vi "Main-PSD+EQP_YCC.vi"() -> ()   [LabVIEW 2014]
uses:
  Main-Stage-Based/(Global) Current handle and LaserPower_YCC.vi
  <vilib>/DAQmx/create/channels.llb/DAQmx Create Channel (AI-Voltage-Basic).vi
  <vilib>/DAQmx/configure/timing.llb/DAQmx Timing (Sample Clock).vi
  <vilib>/DAQmx/read.llb/DAQmx Read (Analog 2D DBL NChan NSamp).vi
panel:
  out "QPD raw(V) xyz":dbl[][](array[numeric])
  out "kx (pN/nm)":dbl
  in  "Who's Data":enum16{"YCC", "PYW", "LCH", "YYH"}(ring)
  in  "Save?":bool
  out "Frequency (Hz)\n0,df, 2df,...(n/2-1)Fs":dbl[](array[numeric])
  in  "Temperature (C)":dbl=22.0
  out "df (freq. resolution) Hz":dbl
  in  "record time per cycle (s)":dbl=0.125
  in  "EQP on?":bool
  out "Beta (V/um)":dbl[](array[numeric])
  out "Varicance (V^2)":dbl[](array[numeric])
  out "y-variance (V)":dbl format="%0.2f"
  out "x-variance (V)":dbl format="%0.2f"
  out "Y-conversion factor (V/um)":dbl
  out "X-conversion factor (V/um)":dbl
  out "EQP-Trap Stiffness (pN/nm)":dbl[](array[numeric])
  out "best fit parameters-y":dbl[](array[numeric])
  out "best fit parameters-z":dbl[](array[numeric])
  out "best fit parameters-x":dbl[](array[numeric])
  in  "Fit z?":bool
  in  "Fit y?":bool
  out "best nonlinear fit PSDz":dbl[](array[numeric])
  out "best nonlinear fit PSDy":dbl[](array[numeric])
  out "best nonlinear fit PSDx":dbl[](array[numeric])
  in  "Custum Fs (Hz)":i32
  in  "Focal shift factor":dbl=1.22
  out "best fit parameters":dbl[][](array[numeric])
  out "kx/kz":dbl
  in  "Freq End Cut":dbl=60000.0
  in  "Freq Strat Cut":dbl=10.0
  out "Trap Stiffness (pN/nm)":dbl[](array[numeric])
  in  "bead height (um)":dbl=2.0
  in  "bead radius (um)":dbl=0.515
  out "PSDz":dbl[](array[numeric])
  out "PSDy":dbl[](array[numeric])
  out "PSDx":dbl[](array[numeric])
  out "Frequency (Hz)\n0,df, 2df,...1/2Fs":dbl[](array[numeric])
  in  "Tab Control":enum32{"PSD x & y", "PSD x & z"}(tab)
  out "PSD x & y":T1(graph)
  out "PSD x & z":T2(graph)
  out "Corner Frequency (Hz)\n(fx,fy,fz)":dbl[](array[numeric])
  in  "Fit Lorentz PSD?":bool=TRUE
  out "Avg. PSD":dbl[][](array[numeric])
  out "# of PSD sum":i32
  in  "# of PSD Avg.":dbl=50.0
  in  "stop to fit":bool
  in  "T=NI made PSD\nF=YCC made PSD":bool
  out "Sampling rate (Hz)":i32
  in  "physical channels":tag="Dev2/ai2, Dev2/ai0, Dev2/ai16"
  in  "Sampling Rate (Hz)":T3(ring)=enum."131072"
  # "Fc=80k for fs=131072Hz"
  # "x"
  # "y"
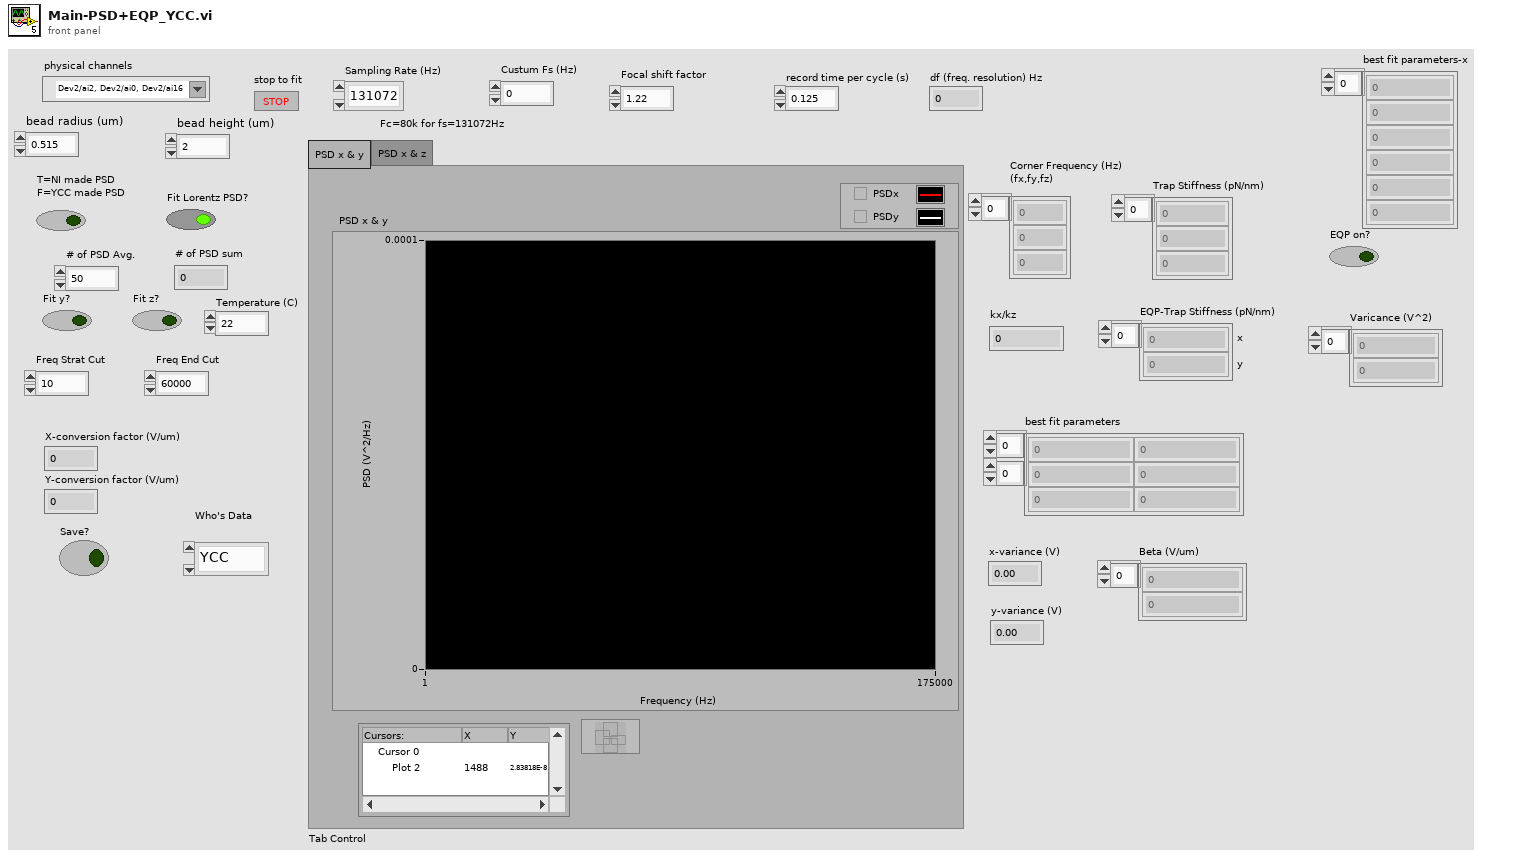
[diagram p1: front panel]
types:
  T1 = cluster{"Frequency (Hz)\ndf, 2df,...1/2Fs":dbl[], "PSDy":dbl[]}[]
  T2 = cluster{"Frequency (Hz)\ndf, 2df,...1/2Fs":dbl[], "PSDz":dbl[]}[]
  T3 = enum16{"custum", "16384", "32768", "65536", "131072", "262144"}
  T4 = cluster{"Frequency (Hz)\n0,df, 2df,...1/2Fs":dbl[], "PSDx":dbl[]}
  T5 = cluster{"Frequency (Hz)\n0,df, 2df,...1/2Fs":dbl[], "PSDz":dbl[]}
  T6 = cluster{"Frequency (Hz)\n0,df, 2df,...1/2Fs":dbl[], "PSDy":dbl[]}
  T7 = cluster{"Frequency (Hz)\n0,df, 2df,...1/2Fs":dbl[], "PSDz":dbl[]}[]
  T8 = cluster{"Frequency (Hz)\n0,df, 2df,...1/2Fs":dbl[], "PSDy":dbl[]}[]
  T9 = cluster{"Frequency (Hz)\n0,df, 2df,...1/2Fs":dbl[], "best nonlinear fit PSDz":dbl[]}
  T10 = cluster{"Frequency (Hz)\n0,df, 2df,...1/2Fs":dbl[], "best nonlinear fit PSDx":dbl[]}
  T11 = cluster{"Frequency (Hz)\n0,df, 2df,...1/2Fs":dbl[], "best nonlinear fit PSDy":dbl[]}
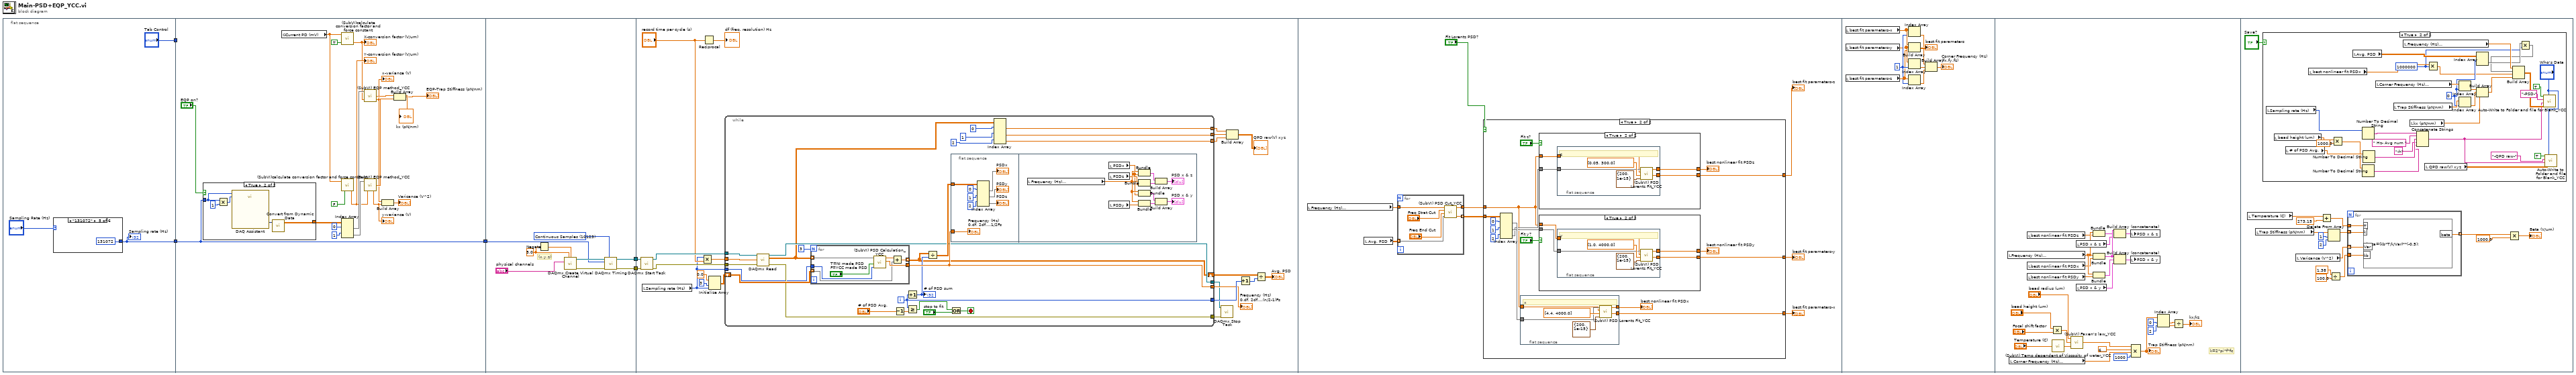
[diagram p0: block diagram]
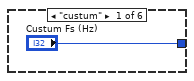
[diagram p2: hidden frame]
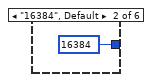
[diagram p3: hidden frame]
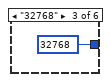
[diagram p4: hidden frame]
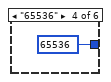
[diagram p5: hidden frame]
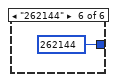
[diagram p6: hidden frame]
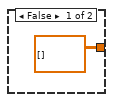
[diagram p7: hidden frame]
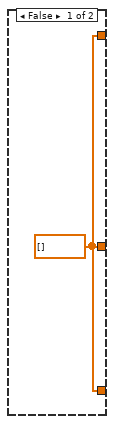
[diagram p8: hidden frame]
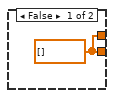
[diagram p9: hidden frame]
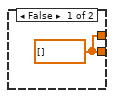
[diagram p10: hidden frame]
diagram:
  n1 = flat-sequence {
    tunnel: [w7] -> w3
    tunnel: ["Tab Control"] -> w1
    tunnel: w3 -> [w32]
    tunnel: [w32] -> w2
    tunnel: w1 -> [_]
    tunnel: w2 -> [w45]
    tunnel: [w42] -> w5
    tunnel: [w41] -> w4
    tunnel: w5 -> [w69]
    tunnel: w4 -> [w68]
    frame #0 {
      n2 = case shown="\"131072\"" "Sampling Rate (Hz)" {
        tunnel: ["Custum Fs (Hz)" 16384 32768 65536 131072 262144] -> w7
        frame "custum" {
        }
        frame "16384", Default {
        }
        frame "32768" {
        }
        frame "65536" {
        }
        frame "131072" {
        }
        frame "262144" {
        }
      }
      "Sampling rate (Hz)" <- w7
    }
    frame #1 {
      n3 = case shown="True" "EQP on?" {
        tunnel: w32 -> [_ w38]
        tunnel: [dbl[][] [] ("Array") w34] -> w21
        frame False {
        }
        frame True {
          n4 = Multiply(x=w38, y=1) -> (x*y=w36:i32)
          n5 = call "DAQ Assistant"("rate"=w38, "number of samples"=w36) -> ("data"=w35:dynamicdata)  [unwired: 15 in, 2 out]
          n6 = call "Convert from Dynamic Data"("Dynamic Data Type"=w35) -> ("Array"=w34:dbl[][])  [unwired: 3 in]
        }
      }
      n7 = global read "(Global) Current handle and LaserPower_YCC.vi" "Current PD (mV)"() -> (w18:dbl)
      n8 = Index Array(array=w21, index (row) #1=0 ("index (row)"), index (row) #2=1 ("index (row)")) -> (element #1=w29:dbl[], element #2=w28:dbl[])  [unwired: 2 in]
      n9 = call "(SubVI)calculate conversion factor and force constant.vi"("X=T\nY=F"=TRUE ("X=T\nY=F"), "laser power (mW)"=w18) -> ("conversion factor (V/um)"=w17:dbl)  [unwired: 2 in, 1 out]
      "X-conversion factor (V/um)" <- w17
      n10 = call "(SubVI)calculate conversion factor and force constant.vi"("X=T\nY=F"=FALSE ("X=T\nY=F"), "laser power (mW)"=w18) -> ("conversion factor (V/um)"=w19:dbl)  [unwired: 2 in, 1 out]
      "Y-conversion factor (V/um)" <- w19
      n11 = call "(SubVI) EQP method_YCC.vi"("Sensitivity (V/um)"=w17, "position (V)"=w29) -> ("variance (V)"=w24:dbl, "k (pN/nm)"=w27:dbl)  [unwired: 2 in]
      "x-variance (V)" <- w24
      "kx (pN/nm)" <- w27
      n12 = call "(SubVI) EQP method_YCC.vi"("Sensitivity (V/um)"=w19, "position (V)"=w28) -> ("variance (V)"=w23:dbl, "k (pN/nm)"=w26:dbl)  [unwired: 2 in]
      "y-variance (V)" <- w23
      n13 = Build Array(w24, w23) -> (→"Varicance (V^2)":dbl[])
      n14 = Build Array(w27, w26) -> (→"EQP-Trap Stiffness (pN/nm)":dbl[])
    }
    frame #2 {
      w40 = 5.0 ("maximum value")
      w43 = 10123 items=["Finite Samples"=10178, "Continuous Samples"=10123, "Hardware Timed Single Point"=12522] ("sample mode")
      # "(x,y,z)"
      n15 = Negate(x=w40) -> (-x=w39:dbl)
      n16 = call-poly <vilib>:"DAQmx Create Virtual Channel.vi"("maximum value"=w40, "minimum value"=w39, "physical channels"="physical channels") -> ("task out"=w46:refnum<k21>, "error out"=w44:errorcluster)  [unwired: 11 in]
      n17 = call-poly <vilib>:"DAQmx Timing.vi"("task/channels in"=w46, "sample mode"=w43, "rate"=w45, "error in"=w44) -> ("task out"=w42:refnum<k21>, "error out"=w41:errorcluster)  [unwired: 10 in]
    }
    frame #3 {
      n18 = call <vilib>:"DAQmx Start Task.vi"("task/channels in"=w69, "error in"=w68) -> ("task out"=w67:refnum<k21>, "error out"=w66:errorcluster)  [unwired: 12 in]
      n19 = local read "Sampling rate (Hz)"() -> (w52:i32)
      n20 = Multiply(x=w52, y="record time per cycle (s)") -> (x*y=w55:dbl)
      n21 = Reciprocal(x="record time per cycle (s)") -> (1/x=→"df (freq. resolution) Hz":dbl)
      n22 = Initialize Array(0.0 ("element"), 3 ("dimension size"), w52) -> (w63:dbl[][])
      n23 = while {
        tunnel: w67 -> [w94]
        tunnel: w66 -> [w93]
        shift-right: [w79] -> w56
        shift-left: w63 -> [w92]
        tunnel: [w83] -> w59
        tunnel: w55 -> [w78]
        tunnel: [w84] -> w62
        tunnel: [w82] -> w58
        tunnel: [w81] -> w57
        tunnel: w52 -> [w77]
        tunnel: [w72] -> w51 mode=concatenating
        tunnel: [w71] -> w50 mode=concatenating
        tunnel: [w70] -> w49 mode=concatenating
        i -> [w84]
        stop <- w87 stop-if-true
        n24 = call-poly <vilib>:"DAQmx Read.vi"("task/channels in"=w94, "number of samples per channel"=w78, "error in"=w93) -> ("task out"=w82:refnum<k21>, "data"=w76:dbl[][], "error out"=w81:errorcluster)  [unwired: 10 in]
        n25 = for {
          N: 3 -> [_]
          tunnel: w76 -> [w119] mode=indexing
          tunnel: w77 -> [w113]
          tunnel: [w116] -> w83
          tunnel: [w115] -> w79 mode=indexing
          tunnel: w92 -> [w114] mode=indexing
          n26 = call "(SubVI) PSD Calculation_YCC.vi"("sampling frequency (Hz)"=w113, "T=NI made PSD\nF=YCC made PSD"="T=NI made PSD\nF=YCC made PSD", "QPD data"=w119) -> ("Frequency (Hz)\n0,df, 2df,...(n/2-1)Fs"=w116:dbl[], "Power Spectrum (V^2 rms) (V^2/Hz)"=w117:dbl[])  [unwired: 3 in]
          n27 = Add(x=w117, y=w114) -> (x+y=w115:dbl[])
        }
        n28 = Decrement(x="# of PSD Avg.") -> (x-1=w89:dbl)
        n29 = Increment(x=w84) -> (x+1=w80:i32)
        "# of PSD sum" <- w80
        n30 = Greater Or Equal?(x=w84, y=w89) -> (x >= y?=w88:bool)
        n31 = Divide(x=w79, y=w80) -> (x/y=w85:dbl[][])
        n32 = Or(x=w88, y="stop to fit") -> (x .or. y?=w87:bool)
        n33 = flat-sequence {
          tunnel: w85 -> [w99]
          tunnel: w83 -> [w96]
          frame #0 {
            n34 = Index Array(array=w99, index (row) #1=0 ("index (row)"), index (row) #2=1 ("index (row)"), index (row) #3=2 ("index (row)")) -> (element #1=→"PSDx":dbl[], element #2=→"PSDy":dbl[], element #3=→"PSDz":dbl[])  [unwired: 3 in]
            "Frequency (Hz)\n0,df, 2df,...1/2Fs" <- w96
          }
          frame #1 {
            n35 = local read "Frequency (Hz)\n0,df, 2df,...1/2Fs"() -> (w108:dbl[])
            n36 = local read "PSDx"() -> (w103:dbl[])
            n37 = local read "PSDz"() -> (w104:dbl[])
            n38 = local read "PSDy"() -> (w109:dbl[])
            n39 = Bundle("Frequency (Hz)\n0,df, 2df,...1/2Fs"=w108, "PSDx"=w103) -> (w106:T4)  [unwired: 1 in]
            n40 = Bundle("Frequency (Hz)\n0,df, 2df,...1/2Fs"=w108, "PSDz"=w104) -> (w105:T5)  [unwired: 1 in]
            n41 = Bundle("Frequency (Hz)\n0,df, 2df,...1/2Fs"=w108, "PSDx"=w103) -> (w110:T4)  [unwired: 1 in]
            n42 = Bundle("Frequency (Hz)\n0,df, 2df,...1/2Fs"=w108, "PSDy"=w109) -> (w111:T6)  [unwired: 1 in]
            n43 = Build Array(w106, w105) -> (→"PSD x & z":T7)
            n44 = Build Array(w110, w111) -> (→"PSD x & y":T8)
          }
        }
        n45 = Index Array(array=w76, index (row) #1=0 ("index (row)"), index (row) #2=1 ("index (row)"), index (row) #3=2 ("index (row)")) -> (element #1=w72:dbl[], element #2=w71:dbl[], element #3=w70:dbl[])  [unwired: 3 in]
      }
      "Frequency (Hz)\n0,df, 2df,...(n/2-1)Fs" <- w59
      n46 = call <vilib>:"DAQmx Stop Task.vi"("task/channels in"=w58, "error in"=w57) -> ()  [unwired: 12 in, 2 out]
      n47 = Build Array(w51, w50, w49) -> (→"QPD raw(V) xyz":dbl[][])
      n48 = Increment(x=w62) -> (x+1=w61:i32)
      n49 = Divide(x=w56, y=w61) -> (x/y=→"Avg. PSD":dbl[][])
    }
    frame #4 {
      n50 = local read "Frequency (Hz)\n0,df, 2df,...(n/2-1)Fs"() -> (w121:dbl[])
      n51 = local read "Avg. PSD"() -> (w120:dbl[][])
      n52 = for {
        tunnel: w120 -> [w133] mode=indexing
        tunnel: w121 -> [w132]
        tunnel: [w131] -> w126
        tunnel: [w130] -> w125 mode=indexing
        n53 = call "(SubVI) PSD Cut_YCC.vi"("PSD"=w133, "Freq End Cut"="Freq End Cut", "Freq Strat Cut"="Freq Strat Cut", "Frequency (Hz)"=w132) -> ("PSD Cut"=w130:dbl[], "Freq Cut"=w131:dbl[])  [unwired: 2 in]
      }
      n54 = case shown="True" "Fit Lorentz PSD?" {
        tunnel: w125 -> [_ w150]
        tunnel: w126 -> [_ w143]
        tunnel: [w134 w138] -> w124
        tunnel: [w134 w137] -> w123
        tunnel: [w134 w136] -> w122
        frame False {
          w134 = dbl[] []
        }
        frame True {
          n55 = Index Array(array=w150, index (row) #1=0 ("index (row)"), index (row) #2=1 ("index (row)"), index (row) #3=2 ("index (row)")) -> (element #1=w146:dbl[], element #2=w145:dbl[], element #3=w144:dbl[])  [unwired: 3 in]
          n56 = flat-sequence {
            tunnel: w146 -> [w176]
            tunnel: w143 -> [w175]
            tunnel: [w174] -> w136
            tunnel: [w173] -> w135
            frame #0 {
              # "x"
              n57 = call "(SubVI) PSD Lorentz Fit_YCC.vi"("termination"=cluster{"max iteration":i32, "tolerance":dbl} {"max iteration"=200, "tolerance"=1e-15}, "initial parameters"=dbl[] [4.4, 4000.0], "Frequency (Hz)"=w175, "PSD (Vrms^2)"=w176) -> ("best fit parameters"=w174:dbl[], "best nonlinear fit PSD"=w173:dbl[])  [unwired: 2 in]
            }
          }
          n58 = case shown="True" "Fit z?" {
            tunnel: w144 -> [_ w155]
            tunnel: w143 -> [_ w154]
            tunnel: [w151 w153] -> w137
            tunnel: [w151 w152] -> w141
            frame False {
              w151 = dbl[] [] ("best nonlinear fit PSD")
            }
            frame True {
              n59 = flat-sequence {
                tunnel: w155 -> [w159]
                tunnel: w154 -> [w158]
                tunnel: [w157] -> w153
                tunnel: [w156] -> w152
                frame #0 {
                  # "z"
                  n60 = call "(SubVI) PSD Lorentz Fit_YCC.vi"("termination"=cluster{"max iteration":i32, "tolerance":dbl} {"max iteration"=200, "tolerance"=1e-15}, "initial parameters"=dbl[] [0.05, 300.0], "Frequency (Hz)"=w158, "PSD (Vrms^2)"=w159) -> ("best fit parameters"=w157:dbl[], "best nonlinear fit PSD"=w156:dbl[])  [unwired: 2 in]
                }
              }
            }
          }
          "best nonlinear fit PSDz" <- w141
          n61 = case shown="True" "Fit y?" {
            tunnel: w145 -> [_ w166]
            tunnel: w143 -> [_ w165]
            tunnel: [w162 w164] -> w138
            tunnel: [w162 w163] -> w142
            frame False {
              w162 = dbl[] [] ("best nonlinear fit PSD")
            }
            frame True {
              n62 = flat-sequence {
                tunnel: w166 -> [w170]
                tunnel: w165 -> [w169]
                tunnel: [w168] -> w164
                tunnel: [w167] -> w163
                frame #0 {
                  # "y"
                  n63 = call "(SubVI) PSD Lorentz Fit_YCC.vi"("termination"=cluster{"max iteration":i32, "tolerance":dbl} {"max iteration"=200, "tolerance"=1e-15}, "initial parameters"=dbl[] [1.0, 4000.0], "Frequency (Hz)"=w169, "PSD (Vrms^2)"=w170) -> ("best fit parameters"=w168:dbl[], "best nonlinear fit PSD"=w167:dbl[])  [unwired: 2 in]
                }
              }
            }
          }
          "best nonlinear fit PSDy" <- w142
          "best nonlinear fit PSDx" <- w135
        }
      }
      "best fit parameters-y" <- w124
      "best fit parameters-z" <- w123
      "best fit parameters-x" <- w122
    }
    frame #5 {
      w185 = 1 ("index")
      n64 = local read "best fit parameters-x"() -> (w186:dbl[])
      n65 = local read "best fit parameters-y"() -> (w184:dbl[])
      n66 = local read "best fit parameters-z"() -> (w183:dbl[])
      n67 = Index Array(array=w186, index=w185) -> (element=w182:dbl)
      n68 = Build Array(w186, w184, w183) -> (→"best fit parameters":dbl[][])
      n69 = Index Array(array=w184, index=w185) -> (element=w181:dbl)
      n70 = Index Array(array=w183, index=w185) -> (element=w180:dbl)
      n71 = Build Array(w182, w181, w180) -> (→"Corner Frequency (Hz)\n(fx,fy,fz)":dbl[])
    }
    frame #6 {
      # "k=2*pi*f*fc"
      n72 = local read "Frequency (Hz)\n0,df, 2df,...1/2Fs"() -> (w210:dbl[])
      n73 = local read "Corner Frequency (Hz)\n(fx,fy,fz)"() -> (w188:dbl[])
      n74 = local read "best nonlinear fit PSDz"() -> (w191:dbl[])
      n75 = local read "best nonlinear fit PSDx"() -> (w193:dbl[])
      n76 = local read "best nonlinear fit PSDy"() -> (w192:dbl[])
      n77 = Multiply(x="bead height (um)", y="Focal shift factor") -> (x*y=w194:dbl)
      n78 = call "(SubVI) Temp dependent of Viscosity of water_YCC.vi"("Temperature (C)"="Temperature (C)") -> ("Viscosity (mPa*s)"=w189:dbl)  [unwired: 4 in]
      n79 = call "(SubVI) Faxen's law_YCC.vi"("viscosity (cP)"=w189, "bead height (um)"=w194, "bead radius (um)"="bead radius (um)") -> ("Faxen's law of friction coefficient (N/(m/s))"=w212:dbl)  [unwired: 2 in]
      n80 = local read "PSD x & z"() -> (w204:T2)
      n81 = local read "PSD x & y"() -> (w203:T1)
      n82 = Bundle("Frequency (Hz)\n0,df, 2df,...1/2Fs"=w210, "best nonlinear fit PSDz"=w191) -> (w206:T9)  [unwired: 1 in]
      n83 = Bundle("Frequency (Hz)\n0,df, 2df,...1/2Fs"=w210, "best nonlinear fit PSDx"=w193) -> (w207:T10)  [unwired: 1 in]
      n84 = Bundle("Frequency (Hz)\n0,df, 2df,...1/2Fs"=w210, "best nonlinear fit PSDy"=w192) -> (w209:T11)  [unwired: 1 in]
      n85 = Build Array (concatenate)(w207, w206, w204) -> (w205:T2)
      n86 = Build Array (concatenate)(w207, w209, w203) -> (w208:T1)
      n87 = local write "PSD x & z"(w205) -> ()
      n88 = local write "PSD x & y"(w208) -> ()
      n89 = Compound Arithmetic op=MULTIPLY(w212, 6.283185307179586, w188, 1000 ("Numeric")) -> (w202:dbl[])
      "Trap Stiffness (pN/nm)" <- w202
      n90 = Index Array(array=w202, index #1=0 ("index"), index #2=2 ("index")) -> (element #1=w199:dbl, element #2=w198:dbl)
      n91 = Divide(x=w199, y=w198) -> (x/y=→"kx/kz":dbl)
    }
    frame #7 {
      n92 = local read "Temperature (C)"() -> (w216:dbl)
      n93 = local read "Trap Stiffness (pN/nm)"() -> (w224:dbl[])
      n94 = case shown="True" "Save?" {
        frame False {
        }
        frame True {
          w250 = 1000000 ("Numeric")
          w257 = 0 ("index (row)")
          n95 = local read "Sampling rate (Hz)"() -> (w245:i32)
          n96 = local read "bead height (um)"() -> (w239:dbl)
          n97 = local read "# of PSD Avg."() -> (w242:dbl)
          n98 = local read "best nonlinear fit PSDx"() -> (w253:dbl[])
          n99 = Multiply(x=w239, y=1000.0) -> (x*y=w237:dbl)
          n100 = local read "Avg. PSD"() -> (w260:dbl[][])
          n101 = Number To Decimal String(number=w245) -> (decimal integer string=w244:string)  [unwired: 1 in]
          n102 = Number To Decimal String(number=w237) -> (decimal integer string=w236:string)  [unwired: 1 in]
          n103 = Number To Decimal String(number=w242) -> (decimal integer string=w241:string)  [unwired: 1 in]
          n104 = local read "Corner Frequency (Hz)\n(fx,fy,fz)"() -> (w258:dbl[])
          n105 = local read "Trap Stiffness (pN/nm)"() -> (w259:dbl[])
          n106 = local read "Frequency (Hz)\n0,df, 2df,...(n/2-1)Fs"() -> (w261:dbl[])
          n107 = local read "kx (pN/nm)"() -> (w240:dbl)
          n108 = Concatenate Strings(w244, " Hz- Avg num " ("string"), w241, "-h" ("string"), w236) -> (w232:string)
          n109 = local read "QPD raw(V) xyz"() -> (w231:dbl[][])
          n110 = Multiply(x=w253, y=w250) -> (x*y=w252:dbl[])
          n111 = Index Array(array=w258, index=w257) -> (element=w256:dbl)
          n112 = Index Array(array=w259, index=w257) -> (element=w255:dbl)
          n113 = Index Array(array=w260, index (row)=w257) -> (element=w251:dbl[])  [unwired: 1 in]
          n114 = Build Array(w256, w255, w240) -> (w254:dbl[])
          n115 = Multiply(x=w251, y=w250) -> (x*y=w249:dbl[])
          n116 = Build Array(w261, w249, w252, w254) -> (w248:dbl[][])
          n117 = call "Auto-Write to Folder and file for Blank_YCC.vi"("Who's Data"="Who's Data", "data to be saved"=w248, "File name add to the end \n(height)"=w232, "Title"="-PSD-", "Save?"=TRUE) -> ()  [unwired: 3 in, 2 out]
          n118 = call "Auto-Write to Folder and file for Blank_YCC.vi"("Who's Data"="Who's Data", "data to be saved"=w231, "File name add to the end \n(height)"=w232, "Title"="-QPD raw-", "Save?"=TRUE) -> ()  [unwired: 3 in, 2 out]
        }
      }
      n119 = local read "Varicance (V^2)"() -> (w220:dbl[])
      n120 = Add(x=w216, y=273.15) -> (x+y=w226:dbl)
      n121 = Delete From Array(array=w224, length=1, index=2) -> (array with subset deleted=w221:dbl[])  [unwired: 1 out]
      n122 = Divide(x=1.38 ("input variable"), y=100.0) -> (x/y=w229:dbl)
      n123 = for {
        tunnel: w229 -> [w266]
        tunnel: w226 -> [w265]
        tunnel: w221 -> [w264] mode=indexing
        tunnel: w220 -> [w263] mode=indexing
        tunnel: [w262] -> w219 mode=indexing
        n124 = formula code="beta=(kb*T/k/Var)**(-0.5);"("T"=w265, "Var"=w263, "kb"=w266, "k"=w264) -> ("beta"=w262:dbl)
      }
      n125 = Multiply(x=w219, y=1000.0) -> (x*y=→"Beta (V/um)":dbl[])
    }
  }
